vi "PickAndPlace_SiOrHB.vi"(0 "Operations":T1={"GoToToolPos"=TRUE, "PickTool"=TRUE, "GoToSenPCB"=TRUE, "PickSiPCB"=TRUE, "GoToBP"=TRUE, "DropTool"=TRUE}, 1 "VacuumStates":path=path "C:/Users/TTUHEP/Documents/LabVIEW/GantryPrograms/Configs/PickPlaceVacuumStates.json", 5 "AssmbType":enum16{"Sensor", "HB"}(ring)=enum."HB", 7 "Zone":enum16{"ZoneA", "ZoneB", "ZoneC", "ZoneD"}(ring), 9 "Position":enum16{"1", "2"}(ring), 11 "Error In":errorcluster) -> (4 "Log":string, 15 "Error Out":errorcluster)   [LabVIEW 2021]
panel:
  out "ZoneBasedFileNameStarting":string
  in  "HB_PositionPartialFileName":string="HB_Position.txt"
  in  "SiPositionPartialFileName":string="Si_Position.txt"
  in  "PUT_PositionPartialFileName":string="PUT_Position.txt"
  in  "AssemblyPositionPartialFileName":string="BP_Position.txt"
  in  "BaseDirectory":string="C:\\Users\\TTUHEP\\Documents\\LabVIEW\\GantryPrograms\\Configs\\"
  out "Assembly_XYZU":dbl[](array[numeric])
  out "PUT_XYZU":dbl[](array[numeric])
  out "PUT rotation":dbl
  in  "FastZDrop":dbl=65.0
  in  "FastZToolPick":dbl=85.0
  in  "FastZSiPCBPick":dbl=65.0
  in  "LineNo":u8
  in  "ZSpeed":dbl=10.0
  in  "XYSpeed":dbl=100.0
  out "SiPCBXYZU":dbl[](array[numeric])
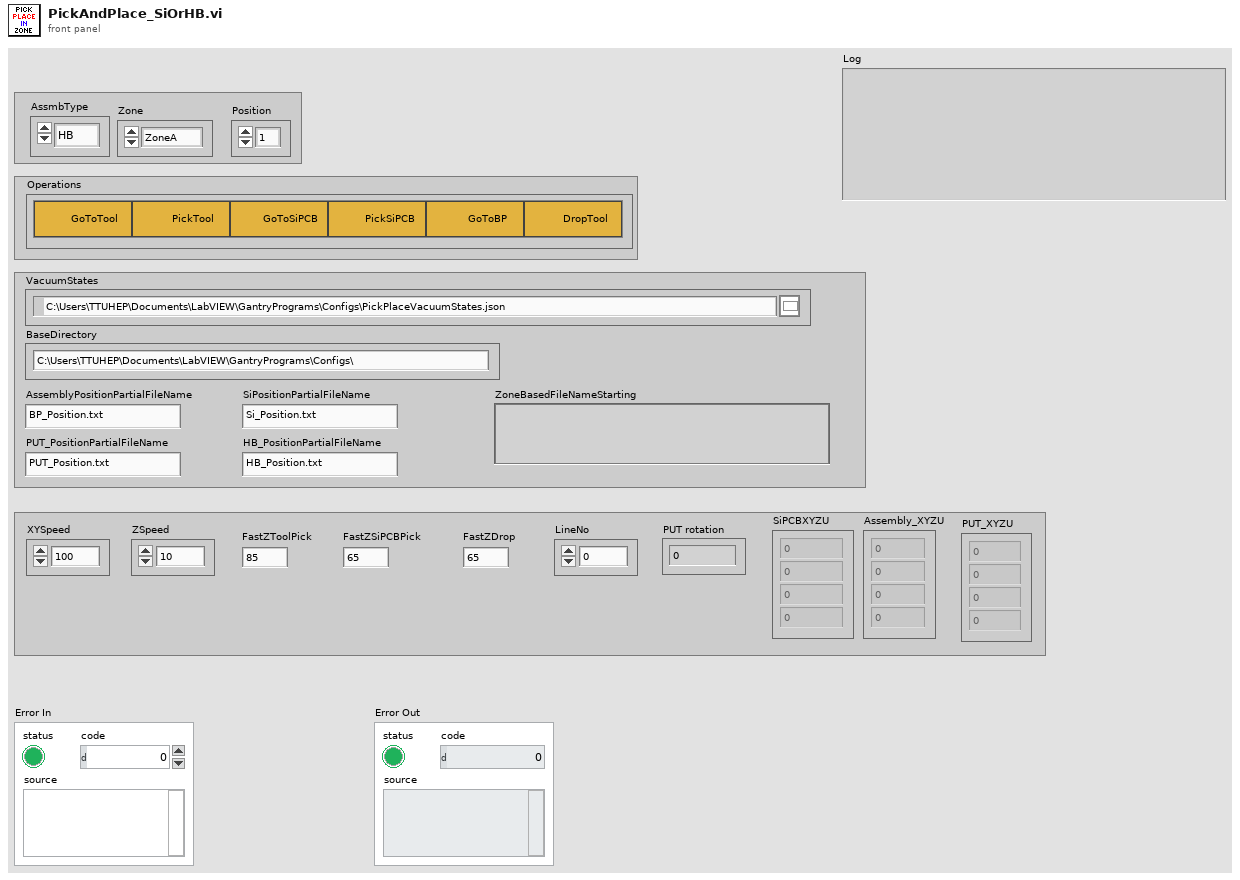
[diagram p1: front panel]
types:
  T1 = cluster{"GoToToolPos":bool, "PickTool":bool, "GoToSenPCB":bool, "PickSiPCB":bool, "GoToBP":bool, "DropTool":bool}
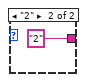
[diagram p2: hidden frame]
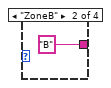
[diagram p3: hidden frame]
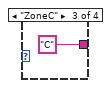
[diagram p4: hidden frame]
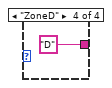
[diagram p5: hidden frame]
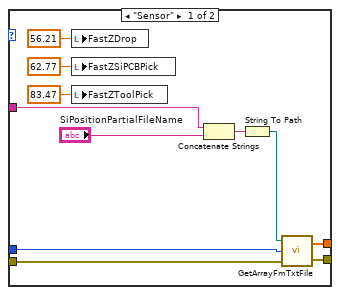
[diagram p6: hidden frame]
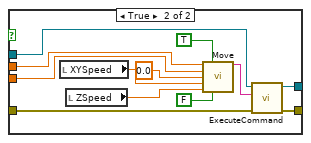
[diagram p7: hidden frame]
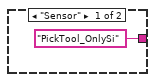
[diagram p9: hidden frame]
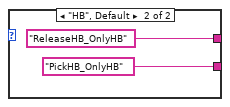
[diagram p12: hidden frame]
diagram:
  n1 = flat-sequence {
    tunnel: [u8 0 ("LineNo")] -> w9
    tunnel: "Zone" -> [w37]
    tunnel: "Position" -> [w36]
    tunnel: [w30] -> w1
    tunnel: [w48] -> w10
    tunnel: w9 -> [w46]
    tunnel: [w46] -> w7
    tunnel: w1 -> [w45]
    tunnel: [w85] -> w29
    tunnel: [w84] -> w28
    tunnel: [w83] -> w27
    tunnel: w10 -> [w81]
    tunnel: w7 -> [w82]
    tunnel: w29 -> [w114]
    tunnel: w28 -> [w113]
    tunnel: w27 -> [w112]
    tunnel: [w111] -> w26
    tunnel: [w110] -> w25
    tunnel: w26 -> [w118]
    tunnel: w25 -> [w117]
    tunnel: [w116] -> w24
    tunnel: [w115] -> w23
    tunnel: w24 -> [w156]
    tunnel: w23 -> [w155]
    tunnel: [w149] -> w22
    tunnel: [w154] -> w21
    tunnel: [w153] -> w20
    tunnel: w22 -> [w182]
    tunnel: w21 -> [w181]
    tunnel: w20 -> [w180]
    tunnel: [w179] -> w19
    tunnel: [w178] -> w18
    tunnel: w19 -> [w186]
    tunnel: w18 -> [w185]
    tunnel: [w184] -> w17
    tunnel: [w183] -> w16
    tunnel: w17 -> [w238]
    tunnel: w16 -> [w237]
    tunnel: [w235] -> w15
    tunnel: [w234] -> w14
    tunnel: [w233] -> w13
    tunnel: w15 -> [w267]
    tunnel: w14 -> [w266]
    tunnel: w13 -> [w264]
    tunnel: [w262] -> w12
    tunnel: [w261] -> w11
    tunnel: w12 -> [w271]
    tunnel: w11 -> [w270]
    tunnel: [w269] -> w5
    tunnel: [w268] -> w4
    tunnel: w5 -> [w312]
    tunnel: w4 -> [w311]
    tunnel: [w310] -> w2
    tunnel: [w315] -> w3
    tunnel: w2 -> [w313]
    frame #0 {
      n2 = case shown="\"ZoneA\", Default" w37 {
        tunnel: ["A" "B" "C" "D"] -> w33
        frame "ZoneA", Default {
        }
        frame "ZoneB" {
        }
        frame "ZoneC" {
        }
        frame "ZoneD" {
        }
      }
      n3 = case shown="\"1\", Default" w36 {
        tunnel: ["1" "2"] -> w32
        frame "1", Default {
        }
        frame "2" {
        }
      }
      n4 = Concatenate Strings(w33, w32, "_" ("string")) -> (w35:string)
      n5 = Concatenate Strings("BaseDirectory", w35) -> (w30:string)
      "ZoneBasedFileNameStarting" <- w30
    }
    frame #1 {
      n6 = case shown="\"HB\", Default" "AssmbType" {
        tunnel: w46 -> [w61 w72]
        tunnel: [w60 w71] -> w50
        tunnel: "Error In" -> [w59 w70]
        tunnel: [w58 w69] -> w48
        tunnel: w45 -> [w53 w65]
        frame "Sensor" {
          n7 = local write "FastZDrop"(56.21 ("FastZDrop")) -> ()
          n8 = local write "FastZSiPCBPick"(62.77 ("FastZSiPCBPick")) -> ()
          n9 = local write "FastZToolPick"(83.47 ("FastZToolPick")) -> ()
          n10 = Concatenate Strings(w53, "SiPositionPartialFileName") -> (w52:string)
          n11 = String To Path(string=w52) -> (path=w51:path)
          n12 = call "GetArrayFmTxtFile.vi"("error in"=w59, "LineNo."=w61, "TextFile"=w51) -> ("error out"=w58:errorcluster, "Array"=w60:dbl[])
        }
        frame "HB", Default {
          n13 = local write "FastZToolPick"(80.0 ("FastZToolPick")) -> ()
          n14 = local write "FastZSiPCBPick"(50.0 ("FastZSiPCBPick")) -> ()
          n15 = local write "FastZDrop"(50.0 ("FastZDrop")) -> ()
          n16 = Concatenate Strings(w65, "HB_PositionPartialFileName") -> (w63:string)
          n17 = String To Path(string=w63) -> (path=w62:path)
          n18 = call "GetArrayFmTxtFile.vi"("error in"=w70, "LineNo."=w72, "TextFile"=w62) -> ("error out"=w69:errorcluster, "Array"=w71:dbl[])
        }
      }
      "SiPCBXYZU" <- w50
    }
    frame #2 {
      n19 = local read "ZoneBasedFileNameStarting"() -> (w77:string)
      n20 = Concatenate Strings(w77, "PUT_PositionPartialFileName") -> (w76:string)
      n21 = String To Path(string=w76) -> (path=w75:path)
      n22 = call "GetArrayFmTxtFile.vi"("error in"=w81, "LineNo."=w82, "TextFile"=w75) -> ("error out"=w74:errorcluster, "Array"=w79:dbl[])
      "PUT_XYZU" <- w79
      n23 = local read "Operations"() -> (w92:T1)
      n24 = call "Connect.vi"("error in (no error)"=w74) -> ("error out"=w73:errorcluster, "controller"=w80:refnum<k24>)  [unwired: 9 in]
      n25 = Index Array(array=w79, index=3) -> (element=w83:dbl)
      "PUT rotation" <- w83
      n26 = Index Array(array=w79, index=0) -> (element=w87:dbl)
      n27 = Index Array(array=w79, index=1) -> (element=w86:dbl)
      n28 = Unbundle By Name(w92) -> ("GoToToolPos"=w91:bool)
      n29 = call "ExecuteCommand.vi"("error in (no error)"=w73, "Command Code"="G90\nG1 Z0 F50", "controller in"=w80) -> ("error out"=w95:errorcluster, "controller out"=w94:refnum<k24>)  [unwired: 6 in, 1 out]
      n30 = case shown="False" w91 {
        tunnel: w94 -> [w97 w106]
        tunnel: w95 -> [w96 w105]
        tunnel: [w96 w104] -> w85
        tunnel: [w97 w103] -> w84
        tunnel: w87 -> [_ w102]
        tunnel: w86 -> [_ w101]
        frame False {
        }
        frame True {
          n31 = local read "XYSpeed"() -> (w99:dbl)
          n32 = local read "ZSpeed"() -> (w98:dbl)
          n33 = call "Move.vi"("X"=w102, "Absolute"=TRUE, "Y"=w101, "Z"=0.0, "SpeedXY (mm/s)"=w99, "SpeedZ (mm/s)"=w98, "Move Z first"=FALSE) -> ("Position Gcode"=w107:string)  [unwired: 8 in]
          n34 = call "ExecuteCommand.vi"("error in (no error)"=w105, "Command Code"=w107, "controller in"=w106) -> ("error out"=w104:errorcluster, "controller out"=w103:refnum<k24>)  [unwired: 6 in, 1 out]
        }
      }
    }
    frame #3 {
      n35 = call "RotateGH_U.vi"("error in (no error)"=w114, "controller in"=w113, "U"=w112) -> ("error out"=w111:errorcluster, "controller out"=w110:refnum<k24>)
    }
    frame #4 {
      n36 = local read "Operations"() -> (w120:T1)
      n37 = Unbundle By Name(w120) -> ("PickTool"=w119:bool)
      n38 = case shown="True" w119 {
        tunnel: w118 -> [w122 w133]
        tunnel: w117 -> [w121 w145]
        tunnel: [w122 w125] -> w116
        tunnel: [w121 w129] -> w115
        frame False {
        }
        frame True {
          w136 = u8 0
          n39 = local read "AssmbType"() -> (w124:enum16{"Sensor", "HB"})
          n40 = case shown="\"HB\", Default" w124 {
            tunnel: ["PickTool_OnlySi" ("ItemName") "PickTool_OnlyHB" ("ItemName")] -> w123
            frame "Sensor" {
            }
            frame "HB", Default {
            }
          }
          n41 = call "JSONfileReader.vi"("error in"=w133, "Variant"=w136, "ItemName"=w123, "FileIn"="VacuumStates") -> ("error out"=w131:errorcluster, "Data"=w135:variant, "Found"=w140:bool)
          n42 = Not(x=w140) -> (.not. x?=w141:bool)
          n43 = Variant To Data(error in=w131, type=w136, Variant=w135) -> (data=w134:u8, error out=w130:errorcluster)
          n44 = local read "FastZToolPick"() -> (w128:dbl)
          n45 = local read "Position"() -> (w144:enum16{"1", "2"})
          n46 = call "AddError.vi"("NoErrorMessage"="Vac OK", "ErrorMessage"="Could not get vacuum state from json file.", "error in"=w130, "code"=-998, "Error?"=w141) -> ("Error out"=w132:errorcluster)  [unwired: 6 in]
          n47 = local read "Zone"() -> (w143:enum16{"ZoneA", "ZoneB", "ZoneC", "ZoneD"})
          n48 = call "ZoneVacCtrldPickDrop.vi"("Position"=w144, "Zone"=w143, "VacuumState"=w134, "error in (no error)"=w132, "controller in"=w145, "Zspeed"=50.0, "Z"=w128) -> ("error out"=w126:errorcluster, "controller out"=w129:refnum<k24>)  [unwired: 3 in]
          n49 = call <vilib>:"Simple Error Handler.vi"("error in (no error)"=w126) -> ("error?"=w127:bool, "error out"=w125:errorcluster)  [unwired: 4 in, 3 out]
          n50 = Stop(stop? (T)=w127) -> ()
        }
      }
    }
    frame #5 {
      n51 = local read "SiPCBXYZU"() -> (w152:dbl[])
      n52 = local read "Operations"() -> (w160:T1)
      n53 = Unbundle By Name(w160) -> ("GoToSenPCB"=w161:bool)
      n54 = local read "PUT rotation"() -> (w151:dbl)
      n55 = Index Array(array=w152, index=3) -> (element=w150:dbl)
      n56 = Index Array(array=w152, index=0) -> (element=w162:dbl)
      n57 = Index Array(array=w152, index=1) -> (element=w163:dbl)
      n58 = Add(x=w151, y=w150) -> (x+y=w149:dbl)
      n59 = case shown="True" w161 {
        tunnel: w155 -> [w165 w174]
        tunnel: w156 -> [w164 w173]
        tunnel: [w164 w172] -> w153
        tunnel: [w165 w171] -> w154
        tunnel: w162 -> [_ w170]
        tunnel: w163 -> [_ w169]
        frame False {
        }
        frame True {
          n60 = local read "XYSpeed"() -> (w166:dbl)
          n61 = local read "ZSpeed"() -> (w167:dbl)
          n62 = call "Move.vi"("X"=w170, "Absolute"=TRUE, "Y"=w169, "Z"=0.0, "SpeedXY (mm/s)"=w166, "SpeedZ (mm/s)"=w167, "Move Z first"=FALSE) -> ("Position Gcode"=w175:string)  [unwired: 8 in]
          n63 = call "ExecuteCommand.vi"("error in (no error)"=w173, "Command Code"=w175, "controller in"=w174) -> ("error out"=w172:errorcluster, "controller out"=w171:refnum<k24>)  [unwired: 6 in, 1 out]
        }
      }
    }
    frame #6 {
      n64 = call "RotateGH_U.vi"("error in (no error)"=w180, "controller in"=w181, "U"=w182) -> ("error out"=w178:errorcluster, "controller out"=w179:refnum<k24>)
    }
    frame #7 {
      n65 = local read "Operations"() -> (w187:T1)
      n66 = Unbundle By Name(w187) -> ("PickSiPCB"=w188:bool)
      n67 = case shown="True" w188 {
        tunnel: w185 -> [w190 w213]
        tunnel: w186 -> [w189 w207]
        tunnel: [w190 w210] -> w183
        tunnel: [w189 w209] -> w184
        frame False {
        }
        frame True {
          w202 = u8 0
          w216 = u8 0
          w195 = "Could not get vacuum state from json file." ("ErrorMessage")
          n68 = local read "AssmbType"() -> (w193:enum16{"Sensor", "HB"})
          n69 = case shown="\"Sensor\"" w193 {
            tunnel: ["PickSi" ("ItemName") "PickHB_OnlyHB" ("ItemName")] -> w192
            tunnel: ["ReleaseSi" ("ItemName") "ReleaseHB_OnlyHB" ("ItemName")] -> w191
            frame "Sensor" {
            }
            frame "HB", Default {
            }
          }
          n70 = local read "VacuumStates"() -> (w198:path)
          n71 = call "JSONfileReader.vi"("error in"=w213, "Variant"=w216, "ItemName"=w192, "FileIn"=w198) -> ("error out"=w212:errorcluster, "Data"=w215:variant, "Found"=w219:bool)
          n72 = Not(x=w219) -> (.not. x?=w220:bool)
          n73 = Variant To Data(error in=w212, type=w216, Variant=w215) -> (data=w214:u8, error out=w211:errorcluster)
          n74 = call "AddError.vi"("NoErrorMessage"="Vac OK", "ErrorMessage"=w195, "error in"=w211, "code"=-998, "Error?"=w220) -> ("Error out"=w197:errorcluster)  [unwired: 6 in]
          n75 = call "JSONfileReader.vi"("error in"=w197, "Variant"=w202, "ItemName"=w191, "FileIn"=w198) -> ("error out"=w200:errorcluster, "Data"=w201:variant, "Found"=w205:bool)
          n76 = Not(x=w205) -> (.not. x?=w206:bool)
          n77 = Variant To Data(error in=w200, type=w202, Variant=w201) -> (data=w194:u8, error out=w199:errorcluster)
          n78 = local read "FastZSiPCBPick"() -> (w208:dbl)
          n79 = local read "Position"() -> (w222:enum16{"1", "2"})
          n80 = call "AddError.vi"("NoErrorMessage"="Vac OK", "ErrorMessage"=w195, "error in"=w199, "code"=-998, "Error?"=w206) -> ("Error out"=w196:errorcluster)  [unwired: 6 in]
          n81 = local read "Zone"() -> (w221:enum16{"ZoneA", "ZoneB", "ZoneC", "ZoneD"})
          n82 = call "ZoneVacCtrldPickDrop_2StepVac.vi"("Position"=w222, "VacuumState2"=w194, "Zone"=w221, "VacuumState1"=w214, "error in (no error)"=w196, "controller in"=w207, "Zspeed"=50.0, "Z"=w208) -> ("error out"=w210:errorcluster, "controller out"=w209:refnum<k24>)  [unwired: 2 in]
        }
      }
    }
    frame #8 {
      n83 = local read "ZoneBasedFileNameStarting"() -> (w231:string)
      n84 = Concatenate Strings(w231, "AssemblyPositionPartialFileName") -> (w229:string)
      n85 = local read "LineNo"() -> (w239:u8)
      n86 = String To Path(string=w229) -> (path=w228:path)
      n87 = local read "Operations"() -> (w246:T1)
      n88 = call "GetArrayFmTxtFile.vi"("error in"=w237, "LineNo."=w239, "TextFile"=w228) -> ("error out"=w236:errorcluster, "Array"=w232:dbl[])
      "Assembly_XYZU" <- w232
      n89 = Unbundle By Name(w246) -> ("GoToBP"=w245:bool)
      n90 = Index Array(array=w232, index=3) -> (element=w233:dbl)
      n91 = Index Array(array=w232, index=0) -> (element=w244:dbl)
      n92 = Index Array(array=w232, index=1) -> (element=w243:dbl)
      n93 = case shown="True" w245 {
        tunnel: w238 -> [w248 w257]
        tunnel: w236 -> [w247 w256]
        tunnel: [w247 w255] -> w235
        tunnel: [w248 w254] -> w234
        tunnel: w244 -> [_ w253]
        tunnel: w243 -> [_ w252]
        frame False {
        }
        frame True {
          n94 = local read "XYSpeed"() -> (w249:dbl)
          n95 = local read "ZSpeed"() -> (w250:dbl)
          n96 = call "Move.vi"("X"=w253, "Absolute"=TRUE, "Y"=w252, "Z"=0.0, "SpeedXY (mm/s)"=w249, "SpeedZ (mm/s)"=w250, "Move Z first"=FALSE) -> ("Position Gcode"=w258:string)  [unwired: 8 in]
          n97 = call "ExecuteCommand.vi"("error in (no error)"=w256, "Command Code"=w258, "controller in"=w257) -> ("error out"=w255:errorcluster, "controller out"=w254:refnum<k24>)  [unwired: 6 in, 1 out]
        }
      }
    }
    frame #9 {
      n98 = local read "PUT rotation"() -> (w265:dbl)
      n99 = Add(x=w265, y=w264) -> (x+y=w263:dbl)
      n100 = call "RotateGH_U.vi"("error in (no error)"=w267, "controller in"=w266, "U"=w263) -> ("error out"=w262:errorcluster, "controller out"=w261:refnum<k24>)
    }
    frame #10 {
      n101 = local read "Operations"() -> (w273:T1)
      n102 = Unbundle By Name(w273) -> ("DropTool"=w272:bool)
      n103 = case shown="True" w272 {
        tunnel: w271 -> [w275 w294]
        tunnel: w270 -> [w274 w293]
        tunnel: [w275 w292] -> w269
        tunnel: [w274 w291] -> w268
        frame False {
        }
        frame True {
          w285 = u8 0
          w300 = u8 0
          n104 = local read "AssmbType"() -> (w276:enum16{"Sensor", "HB"})
          n105 = local read "VacuumStates"() -> (w280:path)
          n106 = case shown="\"HB\", Default" w276 {
            frame "Sensor" {
            }
            frame "HB", Default {
              (unwired) "DropTool" ("ItemName")
              (unwired) "HoldPUT" ("ItemName")
            }
          }
          n107 = call "JSONfileReader.vi"("error in"=w294, "Variant"=w300, "ItemName"="HoldPUT", "FileIn"=w280) -> ("error out"=w307:errorcluster, "Data"=w305:variant, "Found"=w304:bool)
          n108 = Not(x=w304) -> (.not. x?=w303:bool)
          n109 = Variant To Data(error in=w307, type=w300, Variant=w305) -> (data=w306:u8, error out=w308:errorcluster)
          n110 = call "AddError.vi"("NoErrorMessage"="Vac OK", "ErrorMessage"="Could not get vacuum state from json file.", "error in"=w308, "code"=-998, "Error?"=w303) -> ("Error out"=w279:errorcluster)  [unwired: 6 in]
          n111 = call "JSONfileReader.vi"("error in"=w279, "Variant"=w285, "ItemName"="DropTool", "FileIn"=w280) -> ("error out"=w289:errorcluster, "Data"=w288:variant, "Found"=w287:bool)
          n112 = Not(x=w287) -> (.not. x?=w286:bool)
          n113 = Variant To Data(error in=w289, type=w285, Variant=w288) -> (data=w277:u8, error out=w290:errorcluster)
          n114 = local read "FastZDrop"() -> (w309:dbl)
          n115 = local read "Position"() -> (w301:enum16{"1", "2"})
          n116 = call "AddError.vi"("NoErrorMessage"="Vac OK", "ErrorMessage"="Could not get vacuum state from json file.", "error in"=w290, "code"=-998, "Error?"=w286) -> ("Error out"=w278:errorcluster)  [unwired: 6 in]
          n117 = local read "Zone"() -> (w302:enum16{"ZoneA", "ZoneB", "ZoneC", "ZoneD"})
          n118 = call "ZoneVacCtrldPickDrop_2StepVac.vi"("Position"=w301, "VacuumState2"=w277, "Zone"=w302, "VacuumState1"=w306, "error in (no error)"=w278, "controller in"=w293, "Zspeed"=50.0, "Z"=w309) -> ("error out"=w292:errorcluster, "controller out"=w291:refnum<k24>)  [unwired: 2 in]
        }
      }
    }
    frame #11 {
      n119 = call "Disconnect.vi"("error in (no error)"=w312, "controller"=w311) -> ("error out"=w310:errorcluster)  [unwired: 9 in]
    }
    frame #12 {
      n120 = flat-sequence {
        tunnel: [w322] -> w314
        tunnel: w313 -> [w322]
        tunnel: [w325] -> w321
        tunnel: w314 -> [w324]
        tunnel: w321 -> [w333]
        tunnel: [w332] -> w320
        tunnel: [w341] -> w319
        tunnel: w320 -> [w342]
        tunnel: w319 -> [w349]
        tunnel: [w348] -> w318
        tunnel: [w356] -> w317
        tunnel: w318 -> [w356]
        tunnel: [w364] -> w316
        tunnel: w317 -> [w364]
        tunnel: [w372] -> w315
        tunnel: w316 -> [w372]
        frame #0 {
          "Log" <- ""
        }
        frame #1 {
          n121 = local read "AssmbType"() -> (w331:enum16{"Sensor", "HB"})
          n122 = local read "Log"() -> (w326:string)
          n123 = Format Into String(initial string="AssemblyType: ", error in=w324, w331) -> (resulting string=w328:string, error out=w325:errorcluster)  [unwired: 1 in]
          n124 = Concatenate Strings(w326, w328, "\r\n") -> (w330:string)
          n125 = local write "Log"(w330) -> ()
        }
        frame #2 {
          n126 = local read "Zone"() -> (w339:enum16{"ZoneA", "ZoneB", "ZoneC", "ZoneD"})
          n127 = local read "Log"() -> (w336:string)
          n128 = Format Into String(initial string="Zone: ", error in=w333, w339) -> (resulting string=w338:string, error out=w332:errorcluster)  [unwired: 1 in]
          n129 = Concatenate Strings(w336, w338, "\r\n") -> (w337:string)
          n130 = local write "Log"(w337) -> ()
        }
        frame #3 {
          n131 = local read "Position"() -> (w345:enum16{"1", "2"})
          n132 = local read "Log"() -> (w347:string)
          n133 = Format Into String(initial string="AssemblyPosition: ", error in=w342, w345) -> (resulting string=w346:string, error out=w341:errorcluster)  [unwired: 1 in]
          n134 = Concatenate Strings(w347, w346, "\r\n") -> (w340:string)
          n135 = local write "Log"(w340) -> ()
        }
        frame #4 {
          n136 = local read "LineNo"() -> (w355:u8)
          n137 = local read "Log"() -> (w353:string)
          n138 = Format Into String(initial string="ComponentPosTexFileLineNo: ", error in=w349, w355) -> (resulting string=w354:string, error out=w348:errorcluster)  [unwired: 1 in]
          n139 = Concatenate Strings(w353, w354, "\r\n") -> (w352:string)
          n140 = local write "Log"(w352) -> ()
        }
        frame #5 {
          n141 = local read "PUT_XYZU"() -> (w363:dbl[])
          n142 = Array To Spreadsheet String(delimiter (Tab)=",", array=w363, 3:"%f" ("format string")) -> (spreadsheet string=w360:string)
          n143 = local read "Log"() -> (w358:string)
          n144 = Concatenate Strings(w358, "PUT_XYZU: " ("string"), w360) -> (w359:string)
          n145 = local write "Log"(w359) -> ()
        }
        frame #6 {
          n146 = local read "SiPCBXYZU"() -> (w371:dbl[])
          n147 = Array To Spreadsheet String(delimiter (Tab)=",", array=w371, 3:"%f" ("format string")) -> (spreadsheet string=w368:string)
          n148 = local read "Log"() -> (w366:string)
          n149 = Concatenate Strings(w366, "SiPCB_XYZU: " ("string"), w368) -> (w367:string)
          n150 = local write "Log"(w367) -> ()
        }
        frame #7 {
          n151 = local read "Assembly_XYZU"() -> (w373:dbl[])
          n152 = Array To Spreadsheet String(delimiter (Tab)=",", array=w373, 3:"%f" ("format string")) -> (spreadsheet string=w378:string)
          n153 = local read "Log"() -> (w374:string)
          n154 = Concatenate Strings(w374, "Assembly_XYZU: " ("string"), w378) -> (w376:string)
          n155 = local write "Log"(w376) -> ()
        }
      }
    }
  }
  "Error Out" <- w3
